vi "Dialog GraphSetting (Wave).vi"(11 "波形グラフref(in)":refnum<vi>) -> ()   [LabVIEW 2014]
uses:
  TypeDef/GraphSetting Appearance.ctl
  TypeDef/GraphSetting Plot.ctl
  SupportVIs/GraphSetting Scale.ctl
  TypeDef/GraphSetting DisplayFormatType.ctl
  TypeDef/GraphSetting All.ctl
  TypeDef/GraphSetting Command.ctl
  Library/Event/Write User Event (Array).vi
  <vilib>/Utility/xml.llb/Write to XML File(string).vi
  <vilib>/Utility/xml.llb/Read From XML File(string).vi
  <vilib>/measure/NI_MABase.lvlib
panel:
  out "波形グラフ":cluster{dbl, "dt":dbl, "Y":dbl[]}[](graph)
  in  "ファイル読込":bool
  in  "ファイル保存":bool
  in  "タブ制御器":enum32{"外観", "スケール", "プロット"}(tab)
  in  "外観":T1
  in  "Yスケール選択":u16(ring) items=["振幅"]
  in  "スケール(Y軸)":T2
  in  "スケール(X軸)":T2
  in  "Xスケール選択":u16(ring) items=["周波数"]
  in  "プロット":T4 {"Yスケール" items=["振幅"]; "Xスケール" items=["周波数"]; "プロット補間" max=5 step=1; "ポイントスタイル" max=16 step=1; "太さ" max=5 step=1; "ラインスタイル" max=4 step=1}
  in  "プロット選択":u16(ring) items=["プロット0", "プロット1"]
  in  "停止ボタン":bool
  # "スケールのスタイルとカラー"
  # "スケール係数"
  # "スケールのスタイルとカラー"
  # "スケールのスタイルとカラー"
  # "スケール係数"
  # "スケールのスタイルとカラー"
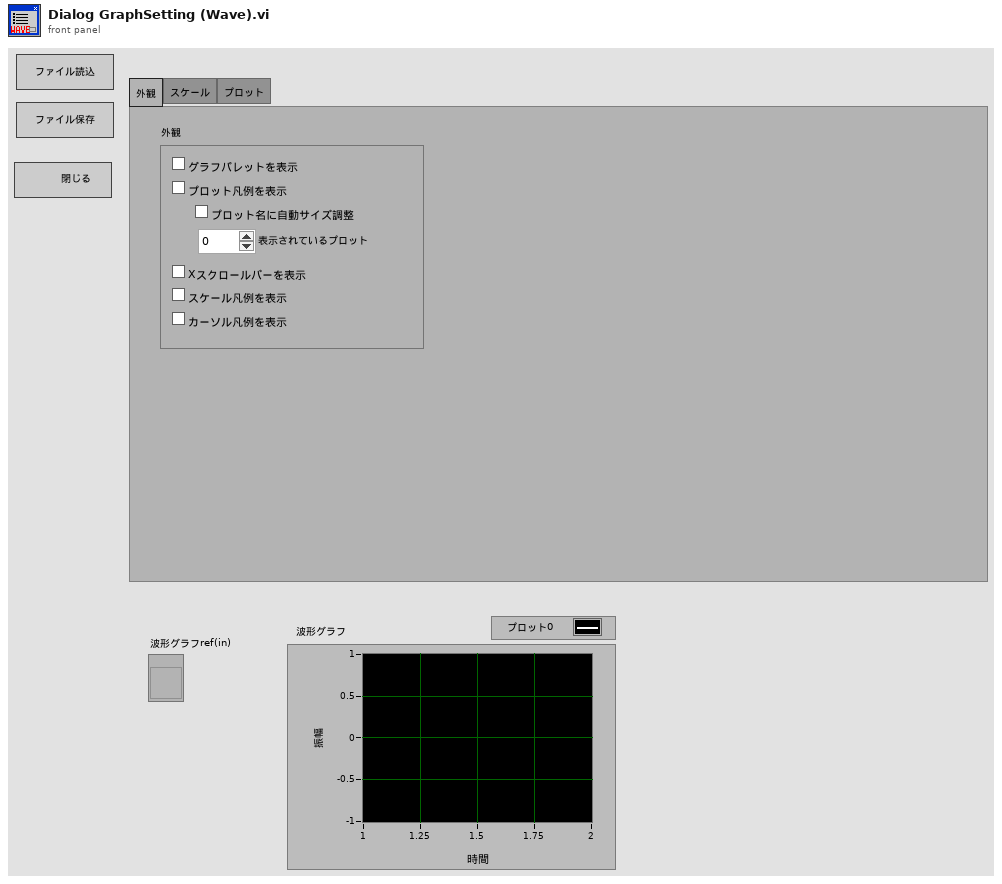
[diagram p1: front panel]
types:
  T1 = typedef "GraphSetting Appearance.ctl" = cluster{"グラフパレットを表示":bool, "プロット凡例を表示":bool, "プロット名に自動サイズ調整":bool, "表示されているプロット":u32, "Xスクロールバーを表示":bool, "スケール凡例を表示":bool, "カーソル凡例を表示":bool}
  T2 = typedef "GraphSetting Scale.ctl" = cluster{"名前":string, "スケールラベルを表示":bool, "スケールを表示":bool, "ログ":bool, "反転":bool, "自動スケール":bool, "最小":dbl, "最大":dbl, "オフセット":dbl, "乗数":dbl, "主目盛り":u32, "補助目盛り":u32, "マーカテキスト":u32, "主グリッド":u32, "補助グリッド":u32, "タイプ":T3, "小数点以下桁数":u8}
  T3 = typedef "GraphSetting DisplayFormatType.ctl" = enum8{"浮動小数点", "科学", "工学", "バイナリ", "８進数", "１６進数", "相対時間", "時間と日時", "SI"}
  T4 = typedef "GraphSetting Plot.ctl" = cluster{"名前":string, "表示":bool, "ラインスタイル":u8, "太さ":u8, "ポイントスタイル":u8, "プロット補間":u8, "ラインカラー":u32, "ポイント/塗りつぶし":u32, "Xスケール":u16, "Yスケール":u16}
  T5 = typedef "GraphSetting All.ctl" = cluster{"外観":T1, "スケールX[]":T2[], "スケールY[]":T2[], "プロット[]":T4[]}
  T6 = typedef "GraphSetting Command.ctl" = enum16{"Get(ref->ctl)", "Set(ctl->ref)"}
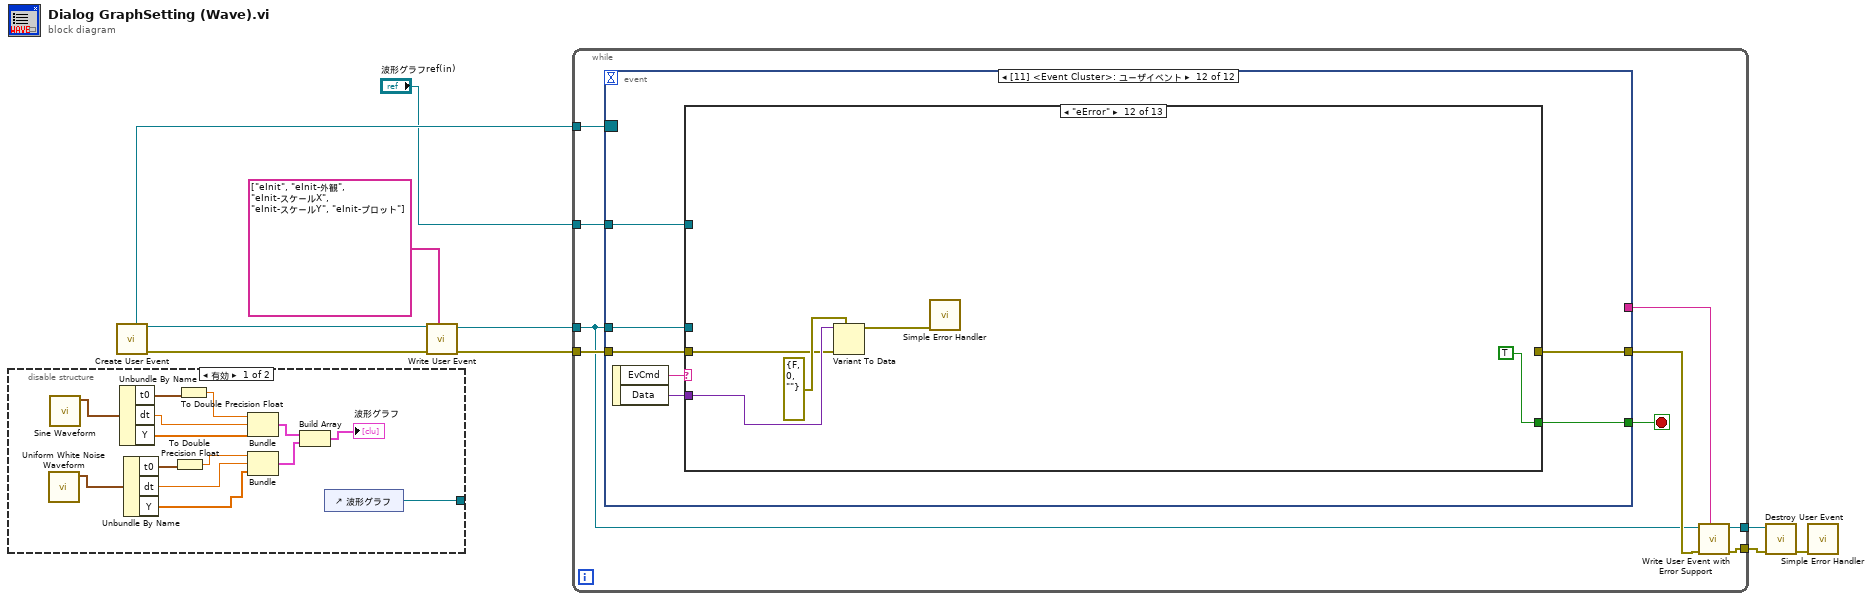
[diagram p0: block diagram]
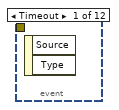
[diagram p3: hidden frame]
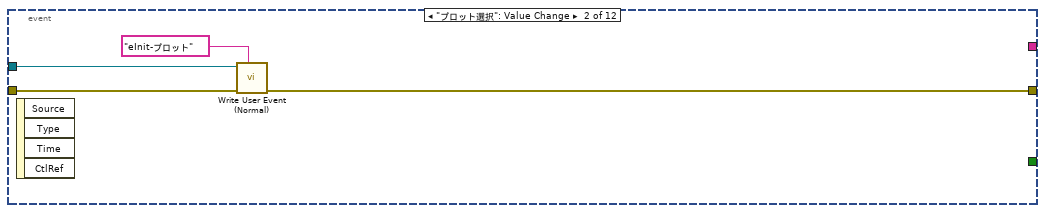
[diagram p4: hidden frame]
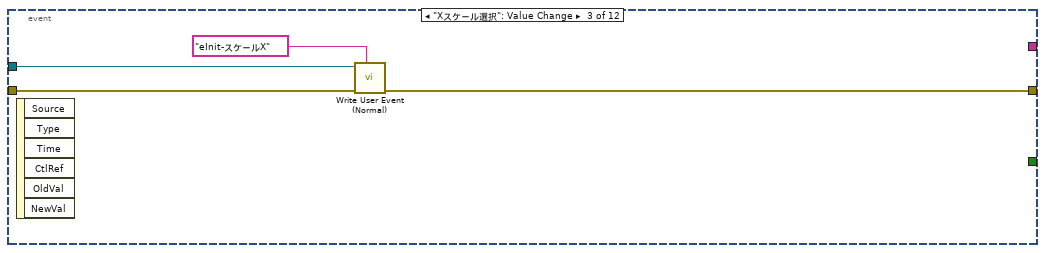
[diagram p5: hidden frame]
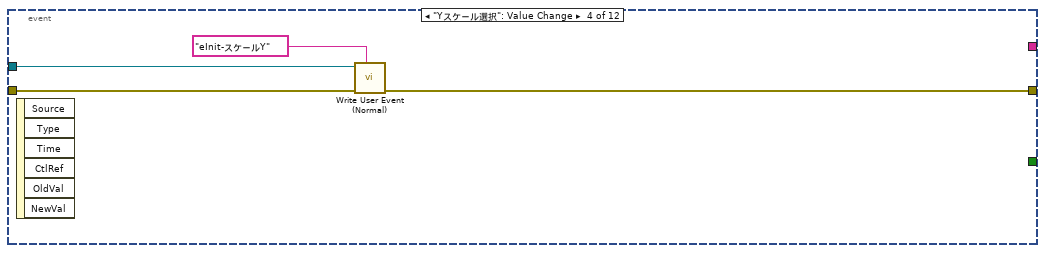
[diagram p6: hidden frame]
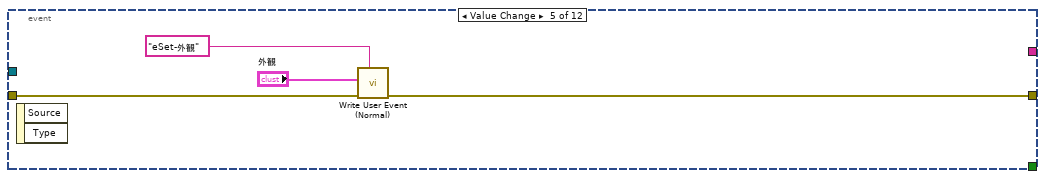
[diagram p7: hidden frame]
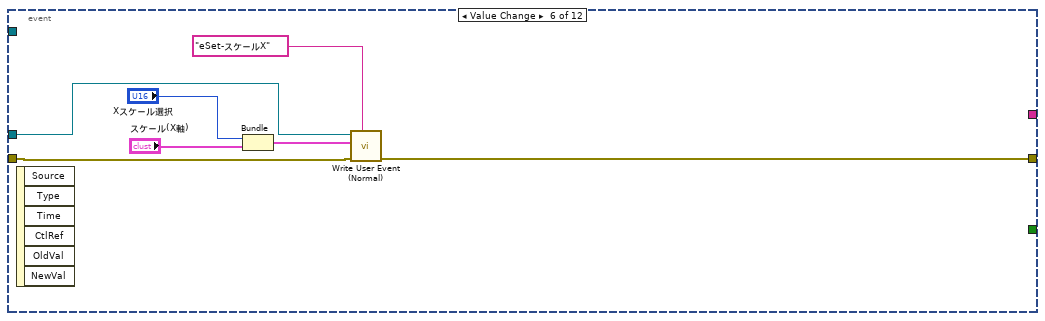
[diagram p8: hidden frame]
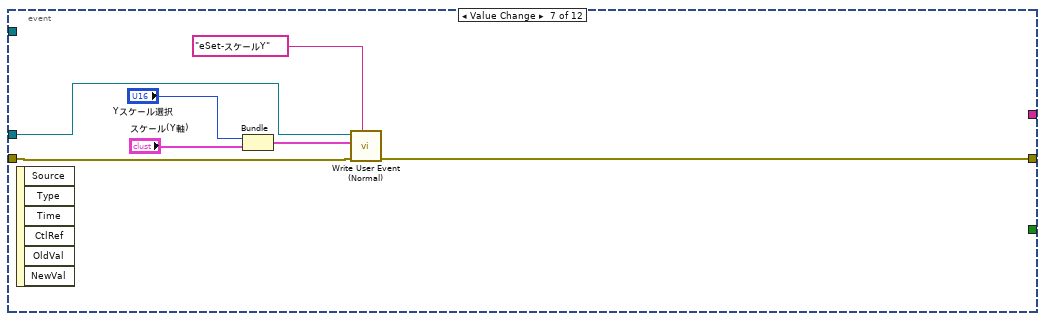
[diagram p9: hidden frame]
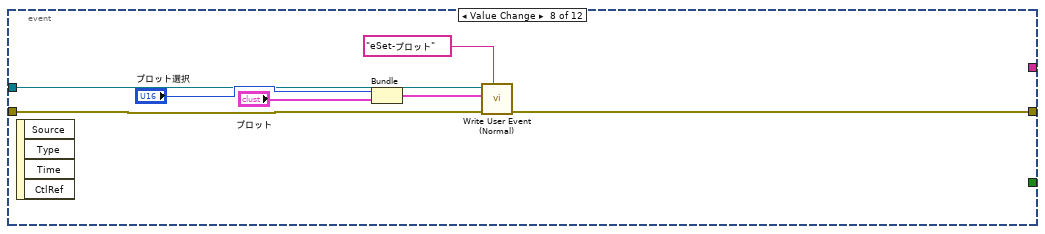
[diagram p10: hidden frame]
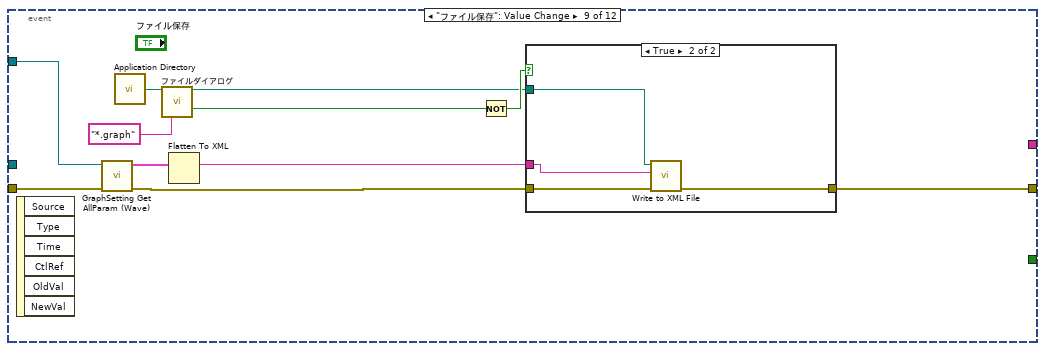
[diagram p11: hidden frame]
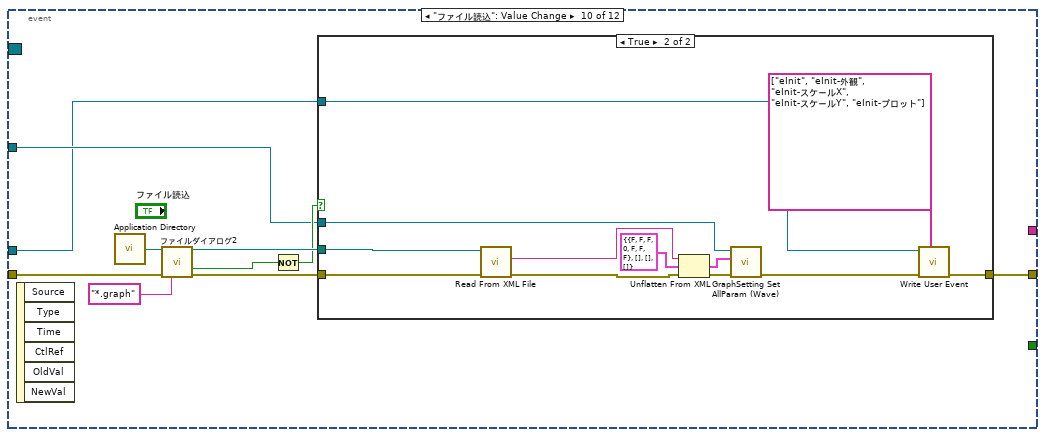
[diagram p13: hidden frame]
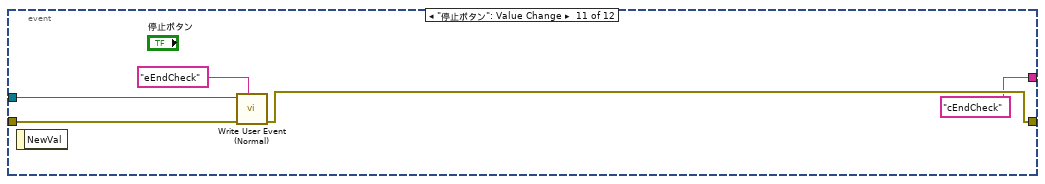
[diagram p15: hidden frame]
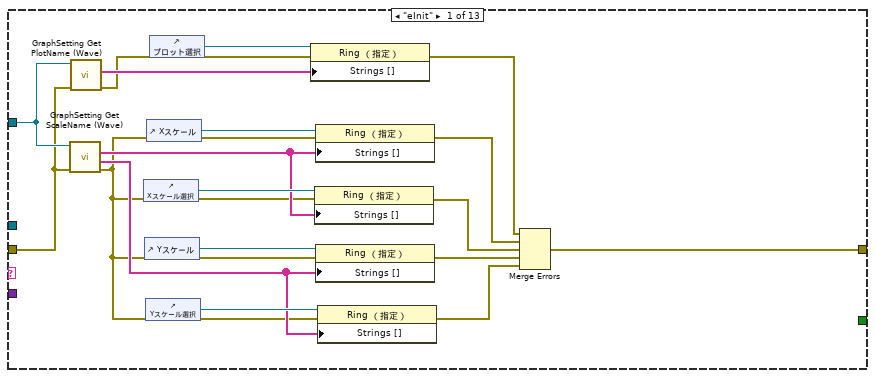
[diagram p16: hidden frame]
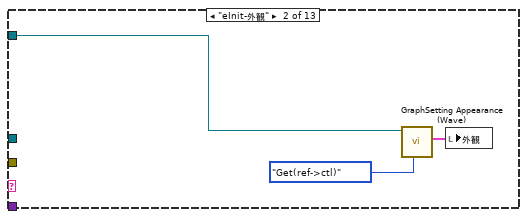
[diagram p17: hidden frame]
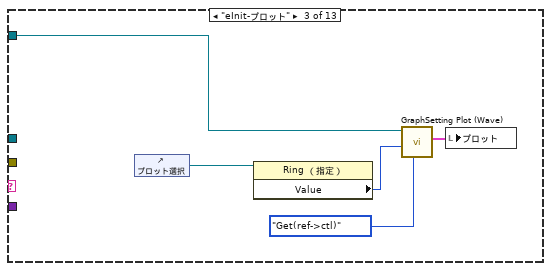
[diagram p18: hidden frame]
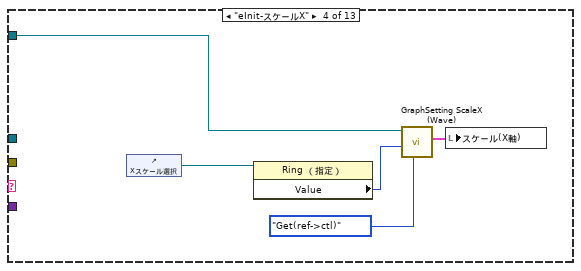
[diagram p19: hidden frame]
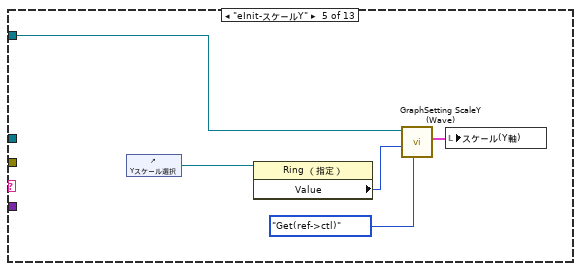
[diagram p20: hidden frame]
diagram:
  n1 = disable-structure shown="有効" {
    disable-tunnel: [w11 _] -> _
    frame Enabled {
      n2 = call <vilib>:"Uniform White Noise Waveform.vi"() -> ("signal out"=w19:waveform(dbl))  [unwired: 10 in, 1 out]
      n3 = call <vilib>:"Sine Waveform.vi"() -> ("signal out"=w24:waveform(dbl))  [unwired: 10 in, 1 out]
      n4 = Unbundle By Name(w24) -> ("t0"=w23:timestamp, "dt"=w21:dbl, "Y"=w20:dbl[])
      n5 = Unbundle By Name(w19) -> ("t0"=w18:timestamp, "dt"=w16:dbl, "Y"=w15:dbl[])
      n6 = To Double Precision Float(number=w18) -> (double precision float=w17:dbl)
      n7 = To Double Precision Float(number=w23) -> (double precision float=w22:dbl)
      n8 = Bundle(w22, "dt"=w21, "Y"=w20) -> (w14:cluster{dbl, "dt":dbl, "Y":dbl[]})  [unwired: 1 in]
      n9 = Bundle(w17, "dt"=w16, "Y"=w15) -> (w13:cluster{dbl, "dt":dbl, "Y":dbl[]})  [unwired: 1 in]
      n10 = Build Array(w14, w13) -> (→"波形グラフ":cluster{dbl, "dt":dbl, "Y":dbl[]}[])
      n11 = control-ref of="波形グラフ"() -> (w11:refnum<vi>)
    }
    frame Disabled {
    }
  }
  n12 = call "Create User Event.vi"() -> ("error out"=w8:errorcluster, "User Event"=w9:refnum<user-event>, "Event Registration Refnum"=w10:refnum<event-registration>)  [unwired: 9 in]
  n13 = call-poly "Write User Event.vi"("EvCmd[]"=string[] ["eInit", "eInit-外観", "eInit-スケールX", "eInit-スケールY", "eInit-プロット"], "エラー入力（エラーなし）"=w8, "ユーザイベント入力"=w9) -> ("エラー出力"=w4:errorcluster, "ユーザイベント出力"=w5:refnum<user-event>)  [unwired: 7 in]
  n14 = while {
    tunnel: w4 -> [w32]
    tunnel: w10 -> [w33]
    tunnel: [w29] -> w7
    tunnel: w5 -> [w25]
    tunnel: "波形グラフref(in)" -> [w31]
    tunnel: [w26] -> w2
    stop <- w27 stop-if-true
    n15 = event shown="[11] <Event Cluster>: ユーザイベント" {
      selector: w33 -> [_ _ _ _ _ _ _ _ _ _ _ _]
      dyn-events: _ -> [_ _ _ _ _ _ _ _ _ _ _ _]
      timeout: _ -> [_ _ _ _ _ _ _ _ _ _ _ _]
      tunnel: [_ _ _ _ _ _ _ _ _ _ _ w117] -> w27
      tunnel: [_ w35 w39 w42 w46 w51 w58 w65 w75 w88 w111 w118] -> w30
      tunnel: w32 -> [_ w36 w41 w44 w47 w50 w59 w66 w72 w94 w113 w119]
      tunnel: w25 -> [_ w37 w40 w43 _ w54 w60 w67 _ w87 w114 w116]
      tunnel: w31 -> [_ _ _ _ _ _ _ _ w71 w89 _ w115]
      tunnel: [_ _ _ _ _ _ _ _ _ _ "cEndCheck" _] -> w28
      event Timeout {
        n16 = event-data() -> ()  [unwired: 1 in, 2 out]
      }
      event "プロット選択": Value Change {
        n17 = event-data() -> ()  [unwired: 1 in, 4 out]
        n18 = call "Write User Event (Normal).vi"("EvCmd"="eInit-プロット", "エラー入力（エラーなし）"=w36, "ユーザイベント入力"=w37) -> ("エラー出力"=w35:errorcluster)  [unwired: 7 in, 1 out]
      }
      event "Xスケール選択": Value Change {
        n19 = event-data() -> ()  [unwired: 1 in, 6 out]
        n20 = call "Write User Event (Normal).vi"("EvCmd"="eInit-スケールX", "エラー入力（エラーなし）"=w41, "ユーザイベント入力"=w40) -> ("エラー出力"=w39:errorcluster)  [unwired: 7 in, 1 out]
      }
      event "Yスケール選択": Value Change {
        n21 = event-data() -> ()  [unwired: 1 in, 6 out]
        n22 = call "Write User Event (Normal).vi"("EvCmd"="eInit-スケールY", "エラー入力（エラーなし）"=w44, "ユーザイベント入力"=w43) -> ("エラー出力"=w42:errorcluster)  [unwired: 7 in, 1 out]
      }
      event Value Change {
        n23 = event-data() -> ()  [unwired: 1 in, 2 out]
        n24 = call "Write User Event (Normal).vi"("EvCmd"="eSet-外観", "エラー入力（エラーなし）"=w47, "データ"="外観") -> ("エラー出力"=w46:errorcluster)  [unwired: 7 in, 1 out]
      }
      event Value Change {
        n25 = event-data() -> ()  [unwired: 1 in, 6 out]
        n26 = Bundle("Xスケール選択"="Xスケール選択", "スケール(X軸)"="スケール(X軸)") -> (w55:cluster{"Xスケール選択":u16, "スケール(X軸)":T2})  [unwired: 1 in]
        n27 = call "Write User Event (Normal).vi"("EvCmd"="eSet-スケールX", "エラー入力（エラーなし）"=w50, "データ"=w55, "ユーザイベント入力"=w54) -> ("エラー出力"=w51:errorcluster)  [unwired: 6 in, 1 out]
      }
      event Value Change {
        n28 = event-data() -> ()  [unwired: 1 in, 6 out]
        n29 = Bundle("Yスケール選択"="Yスケール選択", "スケール(Y軸)"="スケール(Y軸)") -> (w61:cluster{"Yスケール選択":u16, "スケール(Y軸)":T2})  [unwired: 1 in]
        n30 = call "Write User Event (Normal).vi"("EvCmd"="eSet-スケールY", "エラー入力（エラーなし）"=w59, "データ"=w61, "ユーザイベント入力"=w60) -> ("エラー出力"=w58:errorcluster)  [unwired: 6 in, 1 out]
      }
      event Value Change {
        n31 = event-data() -> ()  [unwired: 1 in, 4 out]
        n32 = Bundle("プロット選択"="プロット選択", "プロット"="プロット") -> (w68:cluster{"プロット選択":u16, "プロット":T4})  [unwired: 1 in]
        n33 = call "Write User Event (Normal).vi"("EvCmd"="eSet-プロット", "エラー入力（エラーなし）"=w66, "データ"=w68, "ユーザイベント入力"=w67) -> ("エラー出力"=w65:errorcluster)  [unwired: 6 in, 1 out]
      }
      event "ファイル保存": Value Change {
        n34 = event-data() -> ()  [unwired: 1 in, 6 out]
        n35 = call "GraphSetting Get AllParam (Wave).vi"("エラー入力（エラーなし）"=w72, "波形グラフref(in)"=w71) -> ("エラー出力"=w74:errorcluster, "クラスタ"=w73:cluster{"外観(out)":T1, T2[], T2[], T4[]})  [unwired: 8 in]
        n36 = call <vilib>:"Application Directory.vi"() -> ("Application Directory"=w80:path)
        n37 = call "ファイルダイアログ"("start path"=w80, "pattern (all files)"="*.graph") -> ("selected path"=w76:path, "cancelled"=w77:bool)  [unwired: 10 in, 2 out]
        n38 = Flatten To XML(anything=w73) -> (xml string=w78:string)
        n39 = Not(x=w77) -> (.not. x?=w79:bool)
        n40 = case shown="TRUE" w79 {
          tunnel: w76 -> [_ w86]
          tunnel: w78 -> [_ w85]
          tunnel: w74 -> [w82 w83]
          tunnel: [w82 w84] -> w75
          frame False {
          }
          frame True {
            n41 = call-poly <vilib>:"Write to XML File.vi"("error in (no error)"=w83, "XML Input"=w85, "XML File Path"=w86) -> ("error out"=w84:errorcluster)  [unwired: 6 in, 2 out]
          }
        }
      }
      event "ファイル読込": Value Change {
        n42 = event-data() -> ()  [unwired: 1 in, 6 out]
        n43 = call <vilib>:"Application Directory.vi"() -> ("Application Directory"=w96:path)
        n44 = call "ファイルダイアログ2"("start path"=w96, "error in"=w94, "pattern (all files)"="*.graph") -> ("selected path"=w93:path, "cancelled"=w92:bool, "error out"=w90:errorcluster)  [unwired: 9 in, 1 out]
        n45 = Not(x=w92) -> (.not. x?=w91:bool)
        n46 = case shown="TRUE" w91 {
          tunnel: w93 -> [_ w107]
          tunnel: w90 -> [w97 w105]
          tunnel: w89 -> [_ w102]
          tunnel: [w97 w99] -> w88
          tunnel: w87 -> [_ w101]
          frame False {
          }
          frame True {
            n47 = call-poly <vilib>:"Read From XML File.vi"("error in (no error)"=w105, "XML File Path"=w107) -> ("error out"=w106:errorcluster, "XML Elements"=w108:string)  [unwired: 7 in, 1 out]
            n48 = Unflatten From XML(xml string=w108, type=T5 {"外観"={"グラフパレットを表示"=FALSE, "プロット凡例を表示"=FALSE, "プロット名に自動サイズ調整"=FALSE, "表示されているプロット"=0, "Xスクロールバーを表示"=FALSE, "スケール凡例を表示"=FALSE, "カーソル凡例を表示"=FALSE}, "スケールX[]"=[], "スケールY[]"=[], "プロット[]"=[]} ("出力クラスタ"), error in (no error)=w106) -> (value=w104:T5, error out=w103:errorcluster)
            n49 = call "GraphSetting Set AllParam (Wave).vi"("error in (no error)"=w103, "Chartグラフパラメータ"=w104, "波形グラフref(in)"=w102) -> ("error out"=w100:errorcluster)  [unwired: 8 in]
            n50 = call-poly "Write User Event.vi"("EvCmd[]"=string[] ["eInit", "eInit-外観", "eInit-スケールX", "eInit-スケールY", "eInit-プロット"], "エラー入力（エラーなし）"=w100, "ユーザイベント入力"=w101) -> ("エラー出力"=w99:errorcluster)  [unwired: 7 in, 1 out]
          }
        }
      }
      event "停止ボタン": Value Change {
        n51 = event-data() -> ()  [unwired: 1 in, 1 out]
        n52 = call "Write User Event (Normal).vi"("EvCmd"="eEndCheck", "エラー入力（エラーなし）"=w113, "ユーザイベント入力"=w114) -> ("エラー出力"=w111:errorcluster)  [unwired: 7 in, 1 out]
      }
      event User Event {
        n53 = event-data() -> ("EvCmd"=w121:string, "Data"=w120:variant)  [unwired: 1 in]
        n54 = case shown="\"eError\"" w121 {
          selector: w121 -> [_ _ _ _ _ _ _ _ _ _ _ _ w205]
          tunnel: w120 -> [_ _ _ _ _ w162 w170 w181 w191 _ _ w204 _]
          tunnel: w119 -> [w131 _ _ _ _ w160 w172 w180 w190 w195 w199 w202 _]
          tunnel: [w122 _ _ _ _ w158 w165 w174 w184 w194 w199 _ _] -> w118
          tunnel: [_ _ _ _ _ _ _ _ _ _ TRUE TRUE _] -> w117
          tunnel: w116 -> [_ _ _ _ _ _ _ _ _ w197 _ _ _]
          tunnel: w115 -> [w134 w142 w147 w152 w157 w163 w166 w178 w188 _ _ _ _]
          frame "eInit" {
            n55 = call "GraphSetting Get ScaleName (Wave).vi"("error in (no error)"=w131, "波形グラフref(in)"=w134) -> ("error out"=w128:errorcluster, "Y軸名称[]"=w130:string[], "X軸名称[]"=w137:string[])  [unwired: 7 in]
            n56 = call "GraphSetting Get PlotName (Wave).vi"("error in (no error)"=w131, "波形グラフref(in)"=w134) -> ("error out"=w129:errorcluster, "プロット名称[]"=w132:string[])  [unwired: 8 in]
            n57 = control-ref of="Xスケール選択"() -> (w138:refnum<vi>)
            n58 = control-ref of="Yスケール"() -> (w135:refnum<vi>)
            n59 = control-ref of="Yスケール選択"() -> (w136:refnum<vi>)
            n60 = control-ref of="Xスケール"() -> (w139:refnum<vi>)
            n61 = control-ref of="プロット選択"() -> (w133:refnum<vi>)
            n62 = property class="Ring （指定）"(reference=w133, error in=w129, "Strings []"=w132) -> (error out=w127:errorcluster)  [unwired: 1 out]
            n63 = property class="Ring （指定）"(reference=w138, error in=w128, "Strings []"=w137) -> (error out=w125:errorcluster)  [unwired: 1 out]
            n64 = property class="Ring （指定）"(reference=w139, error in=w128, "Strings []"=w137) -> (error out=w126:errorcluster)  [unwired: 1 out]
            n65 = property class="Ring （指定）"(reference=w135, error in=w128, "Strings []"=w130) -> (error out=w124:errorcluster)  [unwired: 1 out]
            n66 = property class="Ring （指定）"(reference=w136, error in=w128, "Strings []"=w130) -> (error out=w123:errorcluster)  [unwired: 1 out]
            n67 = Merge Errors(w127, w126, w125, w124, w123) -> (w122:errorcluster)
          }
          frame "eInit-外観" {
            n68 = call "GraphSetting Appearance (Wave).vi"("コマンド"=GraphSetting_Command."Get(ref->ctl)", "波形グラフref(in)"=w142) -> ("外観(out)"=w141:T1)  [unwired: 8 in, 1 out]
            n69 = local write "外観"(w141) -> ()
          }
          frame "eInit-プロット" {
            n70 = control-ref of="プロット選択"() -> (w146:refnum<vi>)
            n71 = property class="Ring （指定）"(reference=w146) -> ("Value"=w145:u16)  [unwired: 1 in, 2 out]
            n72 = call "GraphSetting Plot (Wave).vi"("コマンド"=GraphSetting_Command."Get(ref->ctl)", "アクティブプロット"=w145, "波形グラフref(in)"=w147) -> ("プロット(out)"=w143:T4)  [unwired: 7 in, 1 out]
            n73 = local write "プロット"(w143) -> ()
          }
          frame "eInit-スケールX" {
            n74 = control-ref of="Xスケール選択"() -> (w151:refnum<vi>)
            n75 = property class="Ring （指定）"(reference=w151) -> ("Value"=w150:u16)  [unwired: 1 in, 2 out]
            n76 = call "GraphSetting ScaleX (Wave).vi"("コマンド"=GraphSetting_Command."Get(ref->ctl)", "アクティブスケール(X)"=w150, "波形グラフref(in)"=w152) -> ("スケール(out)"=w148:T2)  [unwired: 7 in, 1 out]
            n77 = local write "スケール(X軸)"(w148) -> ()
          }
          frame "eInit-スケールY" {
            n78 = control-ref of="Yスケール選択"() -> (w156:refnum<vi>)
            n79 = property class="Ring （指定）"(reference=w156) -> ("Value"=w155:u16)  [unwired: 1 in, 2 out]
            n80 = call "GraphSetting ScaleY (Wave).vi"("コマンド"=GraphSetting_Command."Get(ref->ctl)", "アクティブスケールY"=w155, "波形グラフref(in)"=w157) -> ("スケール(out)"=w153:T2)  [unwired: 7 in, 1 out]
            n81 = local write "スケール(Y軸)"(w153) -> ()
          }
          frame "eSet-外観" {
            n82 = Variant To Data(error in=w160, Variant=w162) -> (data=w161:T1, error out=w159:errorcluster)  [unwired: 1 in]
            n83 = call "GraphSetting Appearance (Wave).vi"("コマンド"=GraphSetting_Command."Set(ctl->ref)", "error in (no error)"=w159, "外観(in)"=w161, "波形グラフref(in)"=w163) -> ("error out"=w158:errorcluster)  [unwired: 6 in, 1 out]
          }
          frame "eSet-スケールX" {
            n84 = Variant To Data(type=cluster{"Xスケール選択":u16, "スケール(X軸)":T2} {"Xスケール選択"=0, "スケール(X軸)"={"名前"="", "スケールラベルを表示"=FALSE, "スケールを表示"=FALSE, "ログ"=FALSE, "反転"=FALSE, "自動スケール"=FALSE, "最小"=0.0, "最大"=0.0, "オフセット"=0.0, "乗数"=0.0, "主目盛り"=0, "補助目盛り"=0, "マーカテキスト"=0, "主グリッド"=0, "補助グリッド"=0, "タイプ"=enum."浮動小数点", "小数点以下桁数"=0}} ("出力クラスタ"), Variant=w170) -> (data=w169:cluster{"Xスケール選択":u16, "スケール(X軸)":T2})  [unwired: 1 in, 1 out]
            n85 = Unbundle(w169) -> ("Xスケール選択"=w167:u16, "スケール(X軸)"=w168:T2)
            n86 = call "GraphSetting ScaleX (Wave).vi"("コマンド"=GraphSetting_Command."Set(ctl->ref)", "error in (no error)"=w172, "アクティブスケール(X)"=w167, "スケール(in)"=w168, "波形グラフref(in)"=w166) -> ("error out"=w165:errorcluster)  [unwired: 5 in, 1 out]
          }
          frame "eSet-スケールY" {
            n87 = Variant To Data(error in=w180, type=cluster{"Xスケール選択":u16, "スケール(X軸)":T2} {"Xスケール選択"=0, "スケール(X軸)"={"名前"="", "スケールラベルを表示"=FALSE, "スケールを表示"=FALSE, "ログ"=FALSE, "反転"=FALSE, "自動スケール"=FALSE, "最小"=0.0, "最大"=0.0, "オフセット"=0.0, "乗数"=0.0, "主目盛り"=0, "補助目盛り"=0, "マーカテキスト"=0, "主グリッド"=0, "補助グリッド"=0, "タイプ"=enum."浮動小数点", "小数点以下桁数"=0}} ("出力クラスタ"), Variant=w181) -> (data=w179:cluster{"Xスケール選択":u16, "スケール(X軸)":T2}, error out=w175:errorcluster)
            n88 = Unbundle(w179) -> ("Xスケール選択"=w176:u16, "スケール(X軸)"=w177:T2)
            n89 = call "GraphSetting ScaleY (Wave).vi"("コマンド"=GraphSetting_Command."Set(ctl->ref)", "error in (no error)"=w175, "アクティブスケールY"=w176, "スケール(in)"=w177, "波形グラフref(in)"=w178) -> ("error out"=w174:errorcluster)  [unwired: 5 in, 1 out]
          }
          frame "eSet-プロット" {
            n90 = Variant To Data(error in=w190, type=cluster{"プロット選択":u16, "プロット":T4} {"プロット選択"=0, "プロット"={"名前"="", "表示"=FALSE, "ラインスタイル"=0, "太さ"=0, "ポイントスタイル"=0, "プロット補間"=0, "ラインカラー"=0, "ポイント/塗りつぶし"=0, "Xスケール"=0, "Yスケール"=0}} ("出力クラスタ"), Variant=w191) -> (data=w189:cluster{"プロット選択":u16, "プロット":T4}, error out=w187:errorcluster)
            n91 = Unbundle(w189) -> ("プロット選択"=w186:u16, "プロット"=w185:T4)
            n92 = call "GraphSetting Plot (Wave).vi"("コマンド"=GraphSetting_Command."Set(ctl->ref)", "error in (no error)"=w187, "アクティブプロット"=w186, "プロット(in)"=w185, "波形グラフref(in)"=w188) -> ("error out"=w184:errorcluster)  [unwired: 5 in, 1 out]
          }
          frame "eEndCheck" {
            n93 = call "Write User Event (Normal).vi"("EvCmd"="eEnd", "エラー入力（エラーなし）"=w195, "ユーザイベント入力"=w197) -> ("エラー出力"=w194:errorcluster)  [unwired: 7 in, 1 out]
          }
          frame "eEnd" {
          }
          frame "eError" {
            n94 = Variant To Data(error in=w202, type=errorcluster {"status"=FALSE, "code"=0, "source"=""} ("エラー定数"), Variant=w204) -> (data=w201:errorcluster)  [unwired: 1 out]
            n95 = call <vilib>:"Simple Error Handler.vi"("error in (no error)"=w201) -> ()  [unwired: 4 in, 5 out]
          }
          frame Default {
            n96 = call "DialogProgramError.vi"("エラー内容"="ユーザイベント例外" ("エラー詳細"), "エラー詳細"=w205) -> ()  [unwired: 9 in, 1 out]
          }
        }
      }
    }
    n97 = call "Write User Event with Error Support.vi"("EvCmd"=w28, "エラー入力（エラーなし）"=w30, "ユーザイベント入力"=w25) -> ("エラー出力"=w29:errorcluster, "ユーザイベント出力"=w26:refnum<user-event>)  [unwired: 7 in]
  }
  n98 = call "Destroy User Event.vi"("error in (no error)"=w7, "User Event"=w2) -> ("error out"=w6:errorcluster)  [unwired: 9 in]
  n99 = call <vilib>:"Simple Error Handler.vi"("error in (no error)"=w6) -> ()  [unwired: 4 in, 5 out]
